vi "ICR_Hardware_Reset_All.vi"(8 "error in (no error)":errorcluster caption="entrée d'erreur (pas d'erreur)", 10 "STOP ALL":bool, 11 "HARDWARE Resources":T1={"AO6711 Physical Channels"="Analog/ao0:3", "AWG5421 Resource Name"="Waveform", "DIGIT 5122 Resource Name"="Digitizer", "HSDIO Resource Name"="Sequencer"}) -> (0 "error out":errorcluster caption="sortie d'erreur")   [LabVIEW 2015]
uses:
  controls/HARDWARE_Resources.ctl
  <instrlib>/niHSDIO/niHSDIO.llb/niHSDIO_ctl Trigger SW - TrigIdentifier Values (Ring).ctl
  <instrlib>/niHSDIO/niHSDIO.llb/niHSDIO_ctl Trigger SW - TrigName Values (Ring).ctl
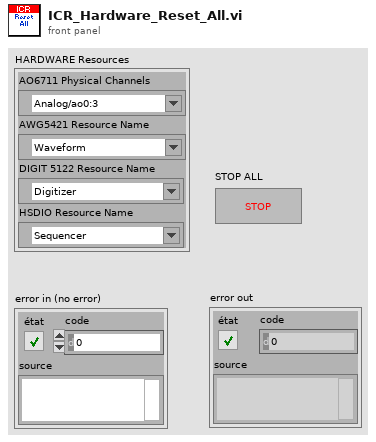
[diagram p1: front panel]
types:
  T1 = typedef "HARDWARE_Resources.ctl" = cluster{"AO6711 Physical Channels":tag, "AWG5421 Resource Name":refnum<k15>, "DIGIT 5122 Resource Name":refnum<k15>, "HSDIO Resource Name":refnum<k15>}
  T2 = typedef "niHSDIO_ctl Trigger SW - TrigIdentifier Values (Ring).ctl" = string
  T3 = typedef "niHSDIO_ctl Trigger SW - TrigName Values (Ring).ctl" = i32
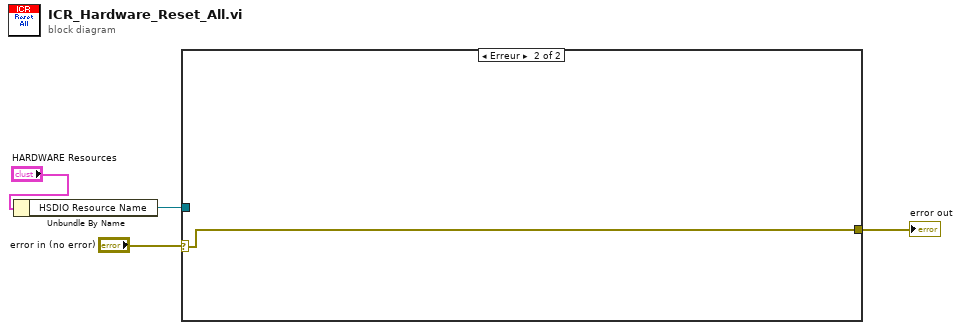
[diagram p0: block diagram]
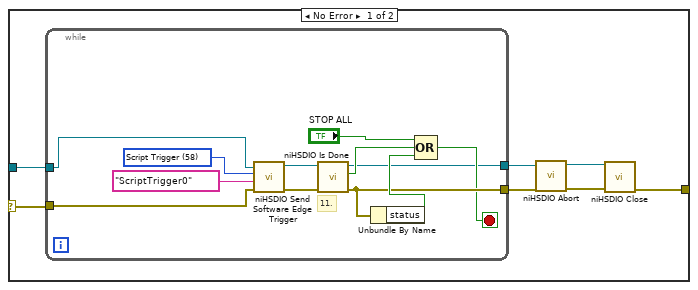
[diagram p2: hidden frame]
diagram:
  n1 = Unbundle By Name("HARDWARE Resources") -> ("HSDIO Resource Name"=w3:refnum<k15>)
  n2 = case shown="Erreur" "error in (no error)" {
    selector: "error in (no error)" -> [w5 w24]
    tunnel: [w11 w24] -> w4
    tunnel: w3 -> [w6 _]
    frame No Error {
      n3 = while {
        tunnel: w5 -> [w23]
        tunnel: w6 -> [w12]
        tunnel: [w17] -> w9
        tunnel: [w15] -> w7
        stop <- w16 stop-if-true
        w13 = T3 58 items=["Start Trigger"=53, "Reference Trigger"=54, "Advance Trigger"=61, "Script Trigger"=58, "Stop Trigger"=82] ("trigger (start trigger)")
        # "11."
        n4 = call <instrlib>:"niHSDIO Send Software Edge Trigger.vi"("error in (no error)"=w23, "trigger identifier (none)"=T2 "ScriptTrigger0", "trigger (start trigger)"=w13, "instrument handle"=w12) -> ("error out"=w21:errorcluster, "instrument handle out"=w22:refnum<k15>)  [unwired: 6 in]
        n5 = call <instrlib>:"niHSDIO Is Done.vi"("error in (no error)"=w21, "instrument handle"=w22) -> ("error out"=w17:errorcluster, "done"=w19:bool, "instrument handle out"=w15:refnum<k15>)  [unwired: 7 in]
        n6 = Unbundle By Name(w17) -> ("status"=w18:bool)
        n7 = Compound Arithmetic op=OR ("Opérateur arithmétique")("STOP ALL", w19, w18) -> (w16:bool)
      }
      n8 = call <instrlib>:"niHSDIO Abort.vi"("error in (no error)"=w9, "instrument handle"=w7) -> ("error out"=w10:errorcluster, "instrument handle out"=w8:refnum<k15>)  [unwired: 8 in]
      n9 = call <instrlib>:"niHSDIO Close.vi"("error in (no error)"=w10, "instrument handle"=w8) -> ("error out"=w11:errorcluster)  [unwired: 9 in]
    }
    frame Error {
    }
  }
  "error out" <- w4
